vi "Destroy Notifiers.vi"(8 "error in (no error)":errorcluster) -> (0 "error out":errorcluster)   [LabVIEW 2017]
uses:
  Reference Action.ctl
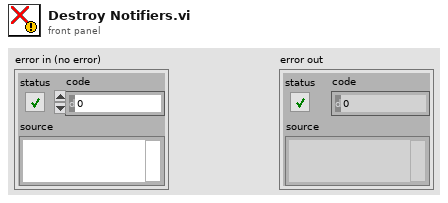
[diagram p1: front panel]
types:
  T1 = typedef "Reference Action.ctl" = enum16{"Set", "Get"}
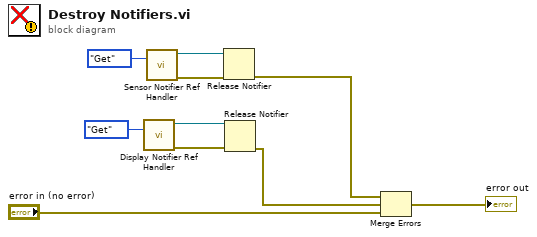
[diagram p0: block diagram]
diagram:
  n1 = call "Display Notifier Ref Handler.vi"("Reference Action"=Reference_Action."Get") -> ("Error Out"=w5:errorcluster, "Notifier Ref Out"=w6:refnum<notifier>)  [unwired: 9 in]
  n2 = call "Sensor Notifier Ref Handler.vi"("Reference Action"=Reference_Action."Get") -> ("Error Out"=w10:errorcluster, "Notifier Ref Out"=w9:refnum<notifier>)  [unwired: 9 in]
  n3 = Release Notifier(notifier=w9, error in (no error)=w10) -> (error out=w4:errorcluster)  [unwired: 1 in, 2 out]
  n4 = Release Notifier(notifier=w6, error in (no error)=w5) -> (error out=w3:errorcluster)  [unwired: 1 in, 2 out]
  n5 = Merge Errors(w4, w3, "error in (no error)") -> (→"error out":errorcluster)
